vi "Publish Data.vi"(6 "Publish Time (Use Current Time)":timestamp, 8 "error in (no error)":errorcluster, 9 "Data to Publish":variant, 10 "Datum Name":string, 11 "IViewModel In":refnum<class "IViewModel.lvclass">) -> (0 "error out":errorcluster, 3 "IViewModel Out":refnum<class "IViewModel.lvclass">)   [LabVIEW 2017, in "IViewModel.lvlib" / "IViewModel.lvclass"]
doc: "<License>\nCopyright © 2017 Composed Systems, LLC | All rights reserved\nwww.composed.io\n\nAuthor: Ethan Stern <ethan.stern@composed.io>\n\nThis software is provided \"AS IS\" WITHOUT WARRANTIES, either express or implied, AND IS FOR EDUCATIONAL PURPOSES ONLY.\n</License>"
uses:
  <vilib>/gpm_packages/@cs/mva-viewable/Source/IViewModel/IViewModel/IViewModel.lvclass
  C:/Program Files/National Instruments/LabVIEW 2017/vi.lib/gpm_packages/@cs/mva-core/Source/IObserver/IObserver/IObserver.lvclass
  <vilib>/gpm_packages/@cs/mva-core/Source/IObserver/IObserver/IObserver.lvclass/IObserver.ctl
  <vilib>/gpm_packages/@cs/mva-viewable/Source/IViewModel/IViewModel/IViewModel.lvclass/IViewModel.ctl
  <vilib>/gpm_packages/@cs/mva-core/Source/IMediator/PublishRequest/PublishRequest.lvclass
  <vilib>/gpm_packages/@cs/mva-core/Source/IMediator/PublishRequest/PublishRequest.lvclass/PublishRequest.ctl
  <vilib>/gpm_packages/@cs/mva-core/Source/IMediator/IMediator Messages/Publish Msg/Publish Msg.lvclass/Publish Msg.ctl
  <vilib>/gpm_packages/@cs/actor-framework-messages/Source/RoundTripMessage/RoundTripMessage.lvclass/RoundTripMessage.ctl
  <vilib>/ActorFramework/Message Enqueuer/Message Enqueuer.lvclass/Message Enqueuer.ctl
  <vilib>/gpm_packages/@cs/actor-framework-messages/Source/RoundTripMessage/Return Round-Trip Message.vi
  <vilib>/ActorFramework/Message Enqueuer/Enqueue.vi
  <vilib>/gpm_packages/@cs/mva-core/Source/IMediator/IMediator Messages/Publish Msg/Publish Msg.lvclass
  C:/Program Files/National Instruments/LabVIEW 2017/vi.lib/gpm_packages/@cs/actor-framework-messages/Source/RoundTripMessage/RoundTripMessage.lvclass
  <vilib>/gpm_packages/@cs/actor-framework-messages/Source/RoundTripMessage/RoundTripMessage.lvclass
  C:/Program Files/National Instruments/LabVIEW 2017/vi.lib/ActorFramework/Message/Message.lvclass
  <vilib>/ActorFramework/Message Priority Queue/Priority Enqueue.vi
  <vilib>/Utility/error.llb/Error Cluster From Error Code.vi
  <vilib>/gpm_packages/@cs/mva-core/Source/IObserver/IObserver/IObserver.lvclass
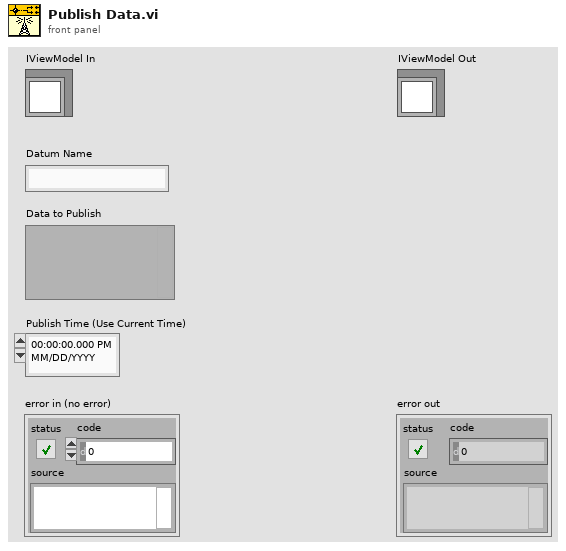
[diagram p1: front panel]
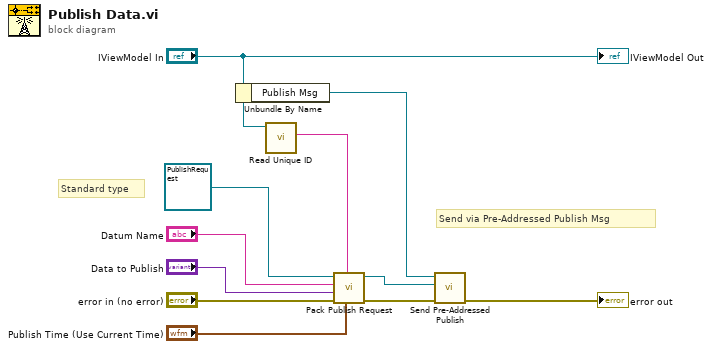
[diagram p0: block diagram]
diagram:
  # "Standard type"
  # "Send via Pre-Addressed Publish Msg"
  n1 = Unbundle By Name("IViewModel In") -> ("Publish Msg"=w11:refnum<class "Publish Msg.lvclass">)
  n2 = call <vilib>:"Read Unique ID.vi"("IObserver In"="IViewModel In") -> ("Unique ID"=w7:string)  [unwired: 10 in]
  n3 = call <vilib>:"Pack Publish Request.vi"("Publication Time (Use Current Time)"="Publish Time (Use Current Time)", "Publisher ID"=w7, "error in (no error)"="error in (no error)", "Value"="Data to Publish", "Datum Name"="Datum Name", "PublishRequest In"=refnum<class "PublishRequest.lvclass"> refnum) -> ("error out"=w5:errorcluster, "PublishRequest Out"=w8:refnum<class "PublishRequest.lvclass">)  [unwired: 4 in]
  n4 = call <vilib>:"Send Pre-Addressed Publish.vi"("error in (no error)"=w5, "PublishRequest"=w8, "Publish Message"=w11) -> ("error out"=→"error out":errorcluster)  [unwired: 8 in]
  "IViewModel Out" <- "IViewModel In"
